vi "BC Windows Main (Test).vi"() -> ()   [LabVIEW 2020]
uses:
  <vilib>/picture/png.llb/Read PNG File.vi
  <vilib>/picture/picture.llb/Draw Flattened Pixmap.vi
  Worker VIs & Controls/Fill Meter.vi
panel:
  in  "Tab Control":enum32{"Main UI", "Setting"}(tab)
  out "HW Status Message":string
  out "Current Beer Picture":picture
  in  "24 Ounces":bool
  in  "16 Ounces":bool
  in  "12 Ounces":bool
  in  "Free Pour":bool
  in  "Stop Pouring":bool
  in  "Shutdown":bool
  out "Filling...":u8(slide) scale=0.0..100.0
  in  "Update Picture":bool
  out "Activity":i32[](listbox)
  in  "Reset Keg":bool
  in  "Change Beer":bool
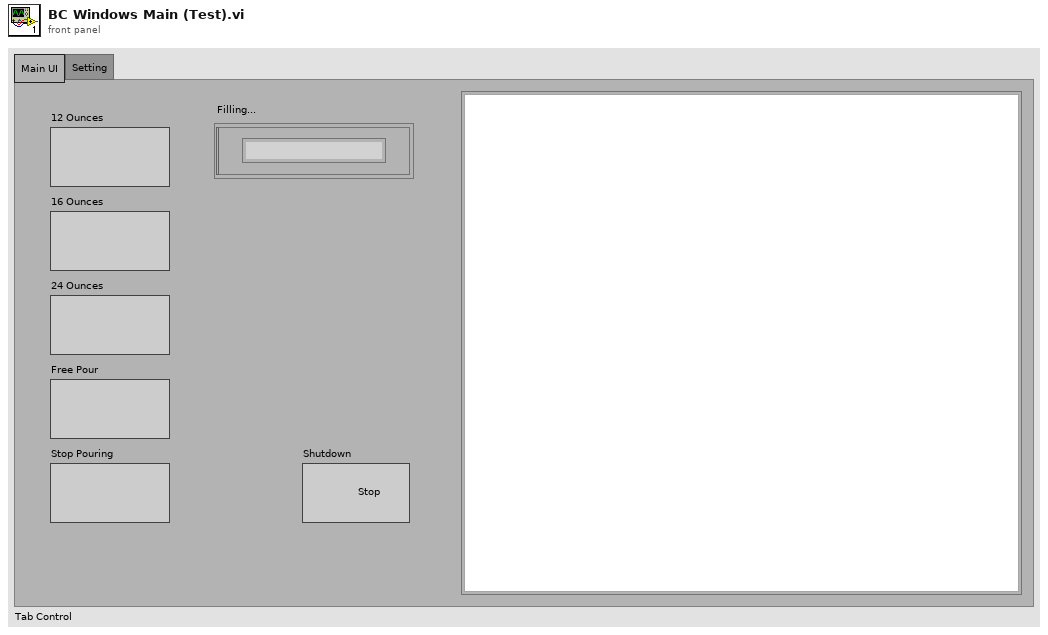
[diagram p1: front panel]
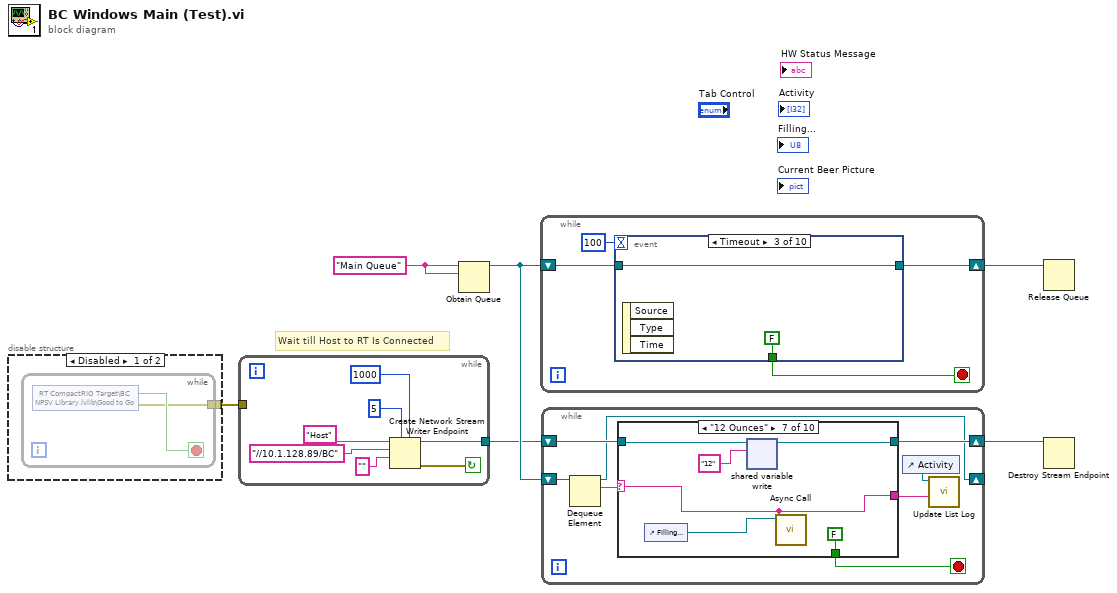
[diagram p0: block diagram]
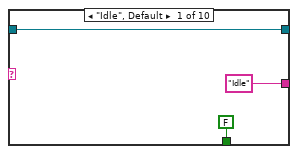
[diagram p3: hidden frame]
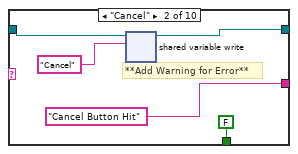
[diagram p4: hidden frame]
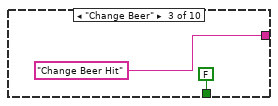
[diagram p5: hidden frame]
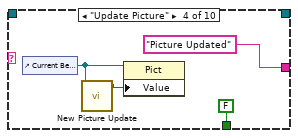
[diagram p6: hidden frame]
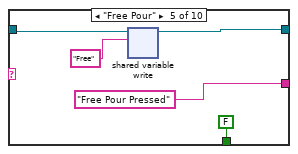
[diagram p7: hidden frame]
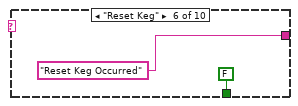
[diagram p8: hidden frame]
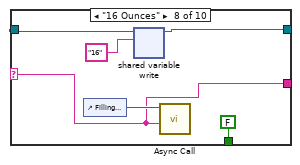
[diagram p9: hidden frame]
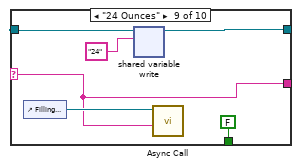
[diagram p10: hidden frame]
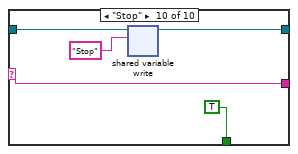
[diagram p11: hidden frame]
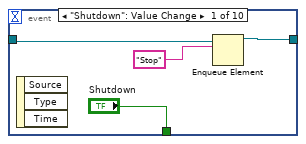
[diagram p12: hidden frame]
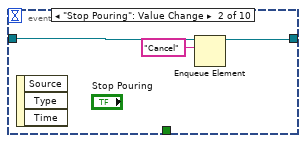
[diagram p13: hidden frame]
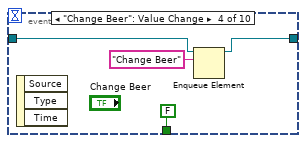
[diagram p14: hidden frame]
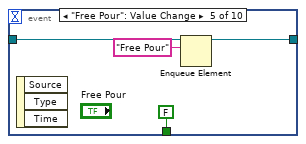
[diagram p15: hidden frame]
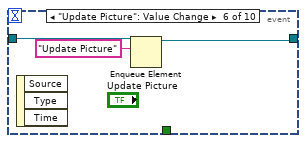
[diagram p16: hidden frame]
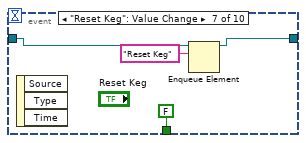
[diagram p17: hidden frame]
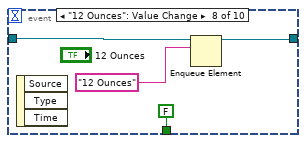
[diagram p18: hidden frame]
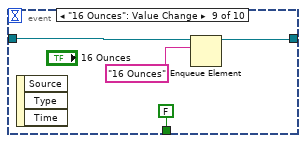
[diagram p19: hidden frame]
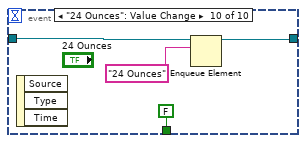
[diagram p20: hidden frame]
diagram:
  w6 = "Main Queue" ("name (unnamed)")
  # "Wait till Host to RT Is Connected"
  n1 = disable-structure shown="Disabled" {
    disable-tunnel: [w7 _] -> w1
    frame Disabled {
      n2 = while {
        tunnel: [w8] -> w7
        stop <- w9 stop-if-true
        n3 = shared-variable "RT CompactRIO Target\\BC NPSV Library.lvlib\\Good to Go"() -> (w9:bool, error out=w8:errorcluster)  [unwired: 1 in]
      }
    }
    frame Enabled {
    }
  }
  n4 = while {
    tunnel: [w15] -> w3
    tunnel: w1 -> [_]
    stop <- w11 continue-if-true
    n5 = Create Network Stream Writer Endpoint(5:1000 ("timeout in ms (-1)"), 7:5 ("writer buffer size"), 9:"" ("writer name"), 10:"//10.1.128.89/BC" ("reader url"), 11:"Host" ("writer name")) -> (0:w11:errorcluster, 3:w15:refnum<k21>)  [unwired: 2 in]
  }
  n6 = Obtain Queue(name (unnamed)=w6, element data type=w6) -> (queue out=w5:refnum<queue>)  [unwired: 3 in, 2 out]
  n7 = while {
    shift-right: [w18] -> w4
    shift-left: w5 -> [w19]
    stop <- w20 stop-if-true
    n8 = event shown="[2] Timeout" {
      selector: _ -> [_ _ _ _ _ _ _ _ _ _]
      dyn-events: _ -> [_ _ _ _ _ _ _ _ _ _]
      timeout: 100 -> [_ _ _ _ _ _ _ _ _ _]
      tunnel: ["Shutdown" _ FALSE ("Stop Button") FALSE ("Stop Button") FALSE ("Stop Button") _ FALSE ("Stop Button") FALSE ("Stop Button") FALSE ("Stop Button") FALSE ("Stop Button")] -> w20
      tunnel: w19 -> [w23 w27 w28 w31 w36 w40 w43 w47 w51 w55]
      tunnel: [w22 w26 w28 w30 w35 w39 w42 w46 w50 w54] -> w18
      event "Shutdown": Value Change {
        n9 = event-data() -> ()  [unwired: 1 in, 3 out]
        n10 = Enqueue Element(queue=w23, element="Stop") -> (queue out=w22:refnum<queue>)  [unwired: 2 in, 2 out]
      }
      event "Stop Pouring": Value Change {
        n11 = event-data() -> ()  [unwired: 1 in, 3 out]
        n12 = Enqueue Element(queue=w27, element="Cancel") -> (queue out=w26:refnum<queue>)  [unwired: 2 in, 2 out]
      }
      event Timeout {
        n13 = event-data() -> ()  [unwired: 1 in, 3 out]
      }
      event "Change Beer": Value Change {
        n14 = event-data() -> ()  [unwired: 1 in, 3 out]
        n15 = Enqueue Element(queue=w31, element="Change Beer") -> (queue out=w30:refnum<queue>)  [unwired: 2 in, 2 out]
      }
      event "Free Pour": Value Change {
        n16 = event-data() -> ()  [unwired: 1 in, 3 out]
        n17 = Enqueue Element(queue=w36, element="Free Pour") -> (queue out=w35:refnum<queue>)  [unwired: 2 in, 2 out]
      }
      event "Update Picture": Value Change {
        n18 = event-data() -> ()  [unwired: 1 in, 3 out]
        n19 = Enqueue Element(queue=w40, element="Update Picture") -> (queue out=w39:refnum<queue>)  [unwired: 2 in, 2 out]
      }
      event "Reset Keg": Value Change {
        n20 = event-data() -> ()  [unwired: 1 in, 3 out]
        n21 = Enqueue Element(queue=w43, element="Reset Keg") -> (queue out=w42:refnum<queue>)  [unwired: 2 in, 2 out]
      }
      event "12 Ounces": Value Change {
        n22 = event-data() -> ()  [unwired: 1 in, 3 out]
        n23 = Enqueue Element(queue=w47, element="12 Ounces") -> (queue out=w46:refnum<queue>)  [unwired: 2 in, 2 out]
      }
      event "16 Ounces": Value Change {
        n24 = event-data() -> ()  [unwired: 1 in, 3 out]
        n25 = Enqueue Element(queue=w51, element="16 Ounces") -> (queue out=w50:refnum<queue>)  [unwired: 2 in, 2 out]
      }
      event "24 Ounces": Value Change {
        n26 = event-data() -> ()  [unwired: 1 in, 3 out]
        n27 = Enqueue Element(queue=w55, element="24 Ounces") -> (queue out=w54:refnum<queue>)  [unwired: 2 in, 2 out]
      }
    }
  }
  n28 = while {
    shift-right: [w58] -> w2
    shift-left: w3 -> [w59]
    shift-right: [w57] -> _
    shift-left: w5 -> [w64]
    stop <- w62 stop-if-true
    n29 = Dequeue Element(queue=w64) -> (queue out=w57:refnum<queue>, element=w63:string)  [unwired: 2 in, 2 out]
    n30 = case shown="\"12 Ounces\"" w63 {
      selector: w63 -> [_ _ _ _ _ _ w89 w95 w101 w107]
      tunnel: [FALSE FALSE FALSE FALSE FALSE FALSE FALSE FALSE FALSE TRUE] -> w62
      tunnel: ["Idle" ("Command to Input") "Cancel Button Hit" ("Command to Input") "Change Beer Hit" ("Command to Input") "Picture Updated" ("Command to Input") "Free Pour Pressed" ("Command to Input") "Reset Keg Occurred" ("Command to Input") w89 w95 w101 w107] -> w60
      tunnel: w59 -> [w65 w70 _ _ w81 _ w88 w93 w99 w105]
      tunnel: [w65 w68 _ _ w80 _ w87 w92 w98 w104] -> w58
      frame "Idle", Default {
      }
      frame "Cancel" {
        # "**Add Warning for Error**"
        n31 = shared-variable-write(w70, "Cancel" ("data in")) -> (w68:refnum<k21>)  [unwired: 2 in, 2 out]
      }
      frame "Change Beer" {
      }
      frame "Update Picture" {
        n32 = control-ref of="Current Beer Picture"() -> (w75:refnum<vi>)
        n33 = call "New Picture Update.vi"("Frame Reference"=w75) -> ("Updated Picture"=w76:picture)  [unwired: 10 in]
        n34 = property class="Pict"(reference=w75, "Value"=w76) -> ()  [unwired: 1 in, 2 out]
      }
      frame "Free Pour" {
        n35 = shared-variable-write(w81, "Free" ("data in")) -> (w80:refnum<k21>)  [unwired: 2 in, 2 out]
      }
      frame "Reset Keg" {
      }
      frame "12 Ounces" {
        n36 = control-ref of="Filling..."() -> (w90:refnum<vi>)
        n37 = shared-variable-write(w88, "12" ("data in")) -> (w87:refnum<k21>)  [unwired: 2 in, 2 out]
        n38 = call "Async Call.vi"("Pour Size"=w89, "Fill Meter Reference"=w90) -> ()  [unwired: 9 in, 1 out]
      }
      frame "16 Ounces" {
        n39 = control-ref of="Filling..."() -> (w96:refnum<vi>)
        n40 = shared-variable-write(w93, "16" ("data in")) -> (w92:refnum<k21>)  [unwired: 2 in, 2 out]
        n41 = call "Async Call.vi"("Pour Size"=w95, "Fill Meter Reference"=w96) -> ()  [unwired: 9 in, 1 out]
      }
      frame "24 Ounces" {
        n42 = control-ref of="Filling..."() -> (w102:refnum<vi>)
        n43 = shared-variable-write(w99, "24" ("data in")) -> (w98:refnum<k21>)  [unwired: 2 in, 2 out]
        n44 = call "Async Call.vi"("Pour Size"=w101, "Fill Meter Reference"=w102) -> ()  [unwired: 9 in, 1 out]
      }
      frame "Stop" {
        n45 = shared-variable-write(w105, "Stop" ("data in")) -> (w104:refnum<k21>)  [unwired: 2 in, 2 out]
      }
    }
    n46 = control-ref of="Activity"() -> (w61:refnum<vi>)
    n47 = call "Update List Log.vi"("Command to Input"=w60, "reference"=w61) -> ()  [unwired: 10 in]
  }
  n48 = Release Queue(queue=w4) -> ()  [unwired: 2 in, 3 out]
  n49 = Destroy Stream Endpoint(11:w2) -> ()  [unwired: 1 in, 1 out]
